vi "fibonacci.vi"() -> ()   [LabVIEW 2021]
panel:
  out "F(n)":dbl
  in  "n":u8
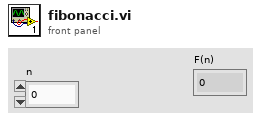
[diagram p1: front panel]
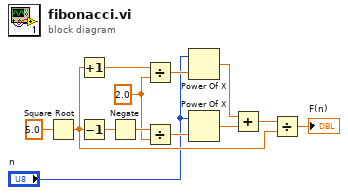
[diagram p0: block diagram]
diagram:
  w8 = 2.0 ("y")
  n1 = Square Root(x=5.0) -> (sqrt(x)=w3:dbl)
  n2 = Increment(x=w3) -> (x+1=w9:dbl)
  n3 = Decrement(x=w3) -> (x-1=w12:dbl)
  n4 = Negate(x=w12) -> (-x=w11:dbl)
  n5 = Divide(x=w9, y=w8) -> (x/y=w7:dbl)
  n6 = Divide(x=w11, y=w8) -> (x/y=w10:dbl)
  n7 = Power Of X(1:w7, 2:"n") -> (0:w5:dbl)
  n8 = Power Of X(1:w10, 2:"n") -> (0:w6:dbl)
  n9 = Add(x=w5, y=w6) -> (x+y=w4:dbl)
  n10 = Divide(x=w4, y=w3) -> (x/y=→"F(n)":dbl)
